vi "CRYOpen Excel.vi"(6 "Numeric":i32, 7 "sActon":string, 8 "error in (no error)":errorcluster, 9 "Excel._Worksheet":refnum<k7>, 10 "Excel._Worksheets":refnum<k7>, 11 "Excel._Application":refnum<k7>) -> (0 "error out":errorcluster, 1 "Excel._Worksheet out":refnum<k7>, 2 "Excel._Worksheets out":refnum<k7>, 3 "Excel._Application out":refnum<k7>)   [LabVIEW 2013]
doc: "This VI opens Excel by creating an Automation Refnum for the Excel.Application object. Next it sets the \"Visible\" property to True/False depending on the Visible input."
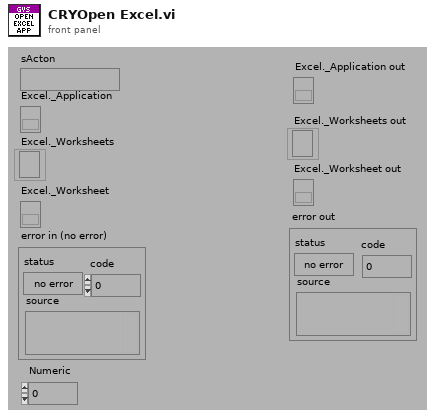
[diagram p1: front panel]
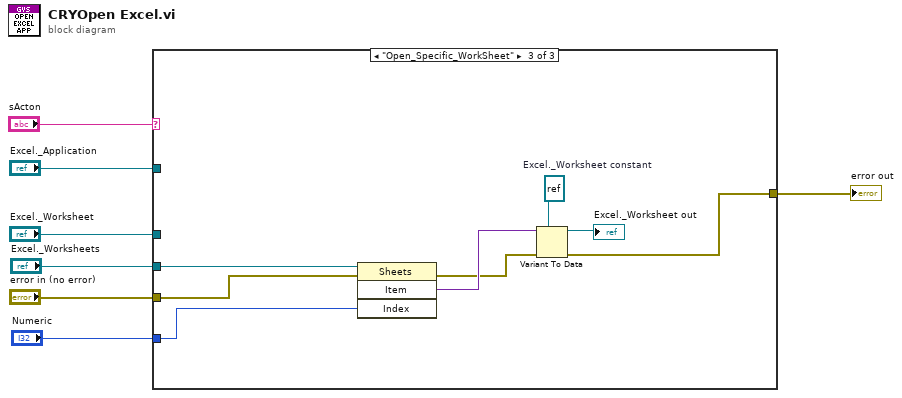
[diagram p0: block diagram]
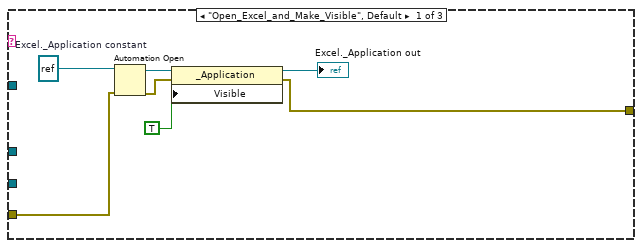
[diagram p2: hidden frame]
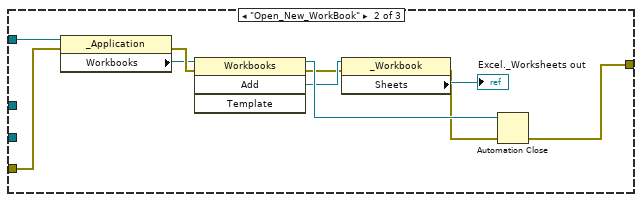
[diagram p3: hidden frame]
diagram:
  n1 = case shown="\"Open_Specific_WorkSheet\"" "sActon" {
    tunnel: "error in (no error)" -> [w12 w20 w30]
    tunnel: [w9 w15 w27] -> w5
    tunnel: "Excel._Application" -> [_ w21 _]
    tunnel: "Excel._Worksheet" -> [_ _ _]
    tunnel: "Numeric" -> [_ _ w25]
    tunnel: "Excel._Worksheets" -> [_ _ w29]
    frame "Open_Excel_and_Make_Visible", Default {
      w8 = refnum<k7> refnum  # Excel._Application constant
      n2 = Automation Open(error in (no error)=w12, Automation Refnum=w8) -> (Automation Refnum=w14:refnum<k7>, error out=w13:errorcluster)  [unwired: 2 out]
      n3 = property class="_Application"(reference=w14, error in=w13, "Visible"=TRUE) -> (reference out=→"Excel._Application out":refnum<k7>, error out=w9:errorcluster)
    }
    frame "Open_New_WorkBook" {
      n4 = property class="_Application"(reference=w21, error in=w20) -> (error out=w23:errorcluster, "Workbooks"=w22:refnum<k7>)  [unwired: 1 out]
      n5 = invoke class="Workbooks" method="Add"(reference=w22, error in=w23) -> (reference out=w24:refnum<k7>, error out=w17:errorcluster, "Add"=w19:refnum<k7>)  [unwired: 2 in, 1 out]
      n6 = property class="_Workbook"(reference=w19, error in=w17) -> (error out=w16:errorcluster, "Sheets"=→"Excel._Worksheets out":refnum<k7>)  [unwired: 1 out]
      n7 = Automation Close(3:w16, 5:w24) -> (0:w15:errorcluster)
    }
    frame "Open_Specific_WorkSheet" {
      w31 = refnum<k7> refnum  # Excel._Worksheet constant
      n8 = invoke class="Sheets" method="Item"(reference=w29, error in=w30, "Index"=w25) -> (error out=w28:errorcluster, "Item"=w32:variant)  [unwired: 1 in, 2 out]
      n9 = Variant To Data(error in=w28, type=w31, Variant=w32) -> (data=→"Excel._Worksheet out":refnum<k7>, error out=w27:errorcluster)
    }
  }
  "error out" <- w5
